vi "set gate shift.vi"(7 "read write":T1, 11 "set gate In":bool=TRUE) -> (3 "set gate out":bool=TRUE)   [LabVIEW 2016]
doc: "determines if the gates are being redrawn or not."
uses:
  controls/read write shift control.ctl
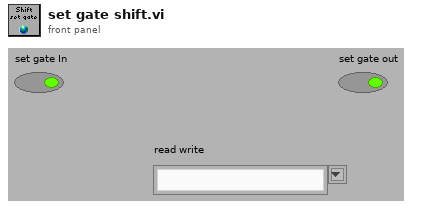
[diagram p1: front panel]
types:
  T1 = typedef "read write shift control.ctl" = string
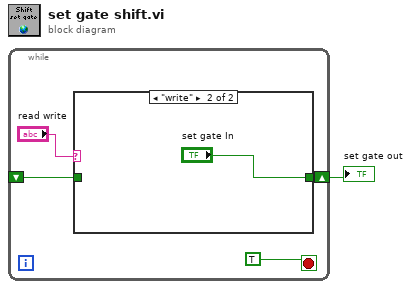
[diagram p0: block diagram]
diagram:
  n1 = while {
    shift-right: [w5] -> w1
    shift-left: _ -> [w3]
    stop <- TRUE ("stop") stop-if-true
    n2 = case shown="\"write\"" "read write" {
      tunnel: [w6 "set gate In"] -> w5
      tunnel: w3 -> [w6 _]
      frame "read", Default {
      }
      frame "write" {
      }
    }
  }
  "set gate out" <- w1
